vi "Puzzle 2-1.vi"() -> ()   [LabVIEW 2022 SP3]
panel:
  out "sum":i32
  out "Array":string[](array[string])
  in  "delimited string":string
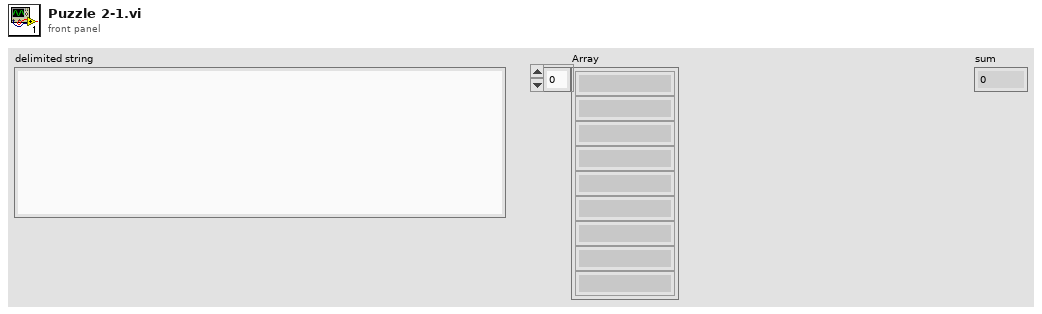
[diagram p1: front panel]
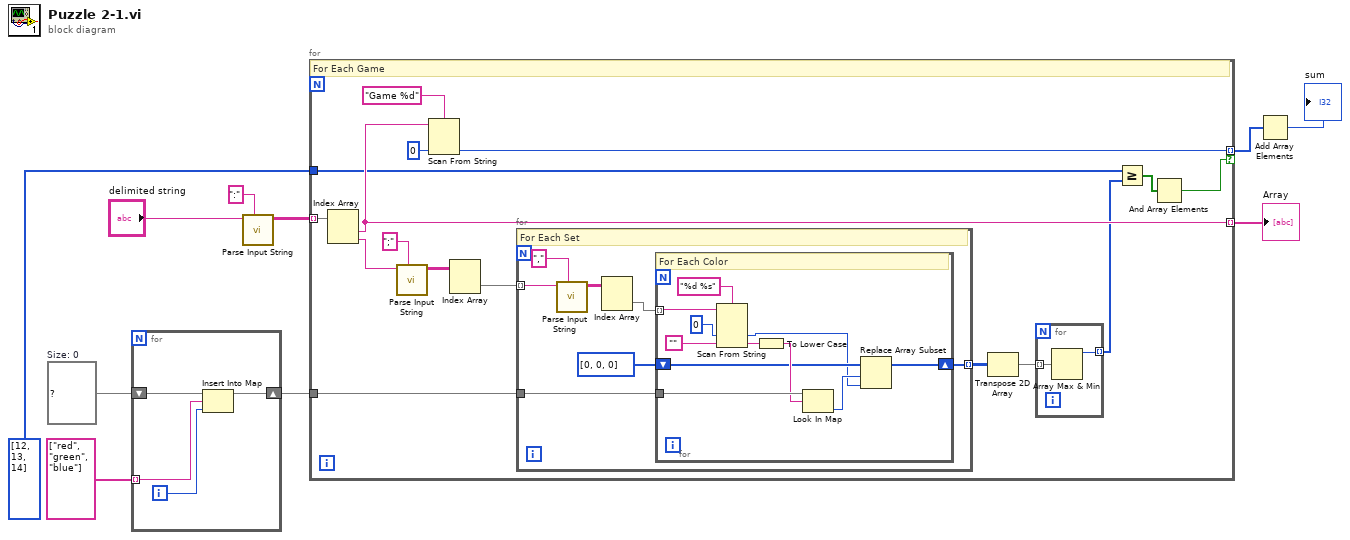
[diagram p0: block diagram]
diagram:
  w6 = map{string, i32} {}  # Size: 0
  n1 = for {
    shift-right: [w12] -> w4
    shift-left: w6 -> [w14]
    tunnel: string[] ["red", "green", "blue"] -> [w13] mode=indexing
    i -> [w11]
    n2 = Insert Into Map(map in=w14, key=w13, value=w11) -> (map out=w12:map{string, i32})  [unwired: 2 out]
  }
  n3 = call "Parse Input String.vi"("delimiter (Tab)"=":", "delimited string"="delimited string") -> ("parsed string"=w8:string[][])  [unwired: 9 in]
  n4 = for {
    tunnel: w8 -> [w29] mode=indexing
    tunnel: [w25] -> w7 mode=indexing
    tunnel: [w22] -> w2 mode=indexing if=w15
    tunnel: w4 -> [w21]
    tunnel: i32[] [12, 13, 14] -> [w18]
    # "For Each Game"
    n5 = Index Array(array=w29) -> (element #1=w25:string, element #2=w28:string)  [unwired: 2 in]
    n6 = call "Parse Input String.vi"("delimiter (Tab)"=";", "delimited string"=w28) -> ("parsed string"=w27:string[][])  [unwired: 9 in]
    n7 = Scan From String(format string="Game %d", input string=w25, default 1=0 ("default value 1")) -> (output 1=w22:i32)  [unwired: 2 in, 3 out]
    n8 = Index Array(array=w27) -> (element=w26:string[])  [unwired: 2 in]
    n9 = for {
      tunnel: w26 -> [w38] mode=indexing
      tunnel: w21 -> [w34]
      tunnel: [w33] -> w20 mode=indexing
      # "For Each Set"
      n10 = call "Parse Input String.vi"("delimiter (Tab)"=",", "delimited string"=w38) -> ("parsed string"=w37:string[][])  [unwired: 9 in]
      n11 = Index Array(array=w37) -> (element=w36:string[])  [unwired: 2 in]
      n12 = for {
        tunnel: w36 -> [w49] mode=indexing
        shift-right: [w40] -> w33
        shift-left: i32[] [0, 0, 0] -> [w43]
        tunnel: w34 -> [w45]
        # "For Each Color"
        n13 = Scan From String(format string="%d %s", input string=w49, default 1=0 ("default value 1"), default 2="" ("default value 2")) -> (output 1=w41:i32, output 2=w46:string)  [unwired: 2 in, 3 out]
        n14 = To Lower Case(string=w46) -> (all lower case string=w44:string)
        n15 = Look In Map(map=w45, key=w44) -> (value=w42:i32)  [unwired: 1 in, 1 out]
        n16 = Replace Array Subset(array=w43, new element=w41, index=w42) -> (w40:i32[])
      }
    }
    n17 = Transpose 2D Array(2D array=w20) -> (transposed array=w19:i32[][])
    n18 = for {
      tunnel: w19 -> [w32] mode=indexing
      tunnel: [w31] -> w17 mode=indexing
      n19 = Array Max & Min(array=w32) -> (max value=w31:i32)  [unwired: 3 out]
    }
    n20 = Greater Or Equal?(x=w18, y=w17) -> (x >= y?=w16:bool[])
    n21 = And Array Elements(Boolean array=w16) -> (logical AND=w15:bool)
  }
  "Array" <- w7
  n22 = Add Array Elements(numeric array=w2) -> (sum=→"sum":i32)
